vi "Main.vi"(8 "error in":errorcluster, 11 "gui in":refnum<class "gui.lvclass">) -> (0 "error out":errorcluster, 3 "gui out":refnum<class "gui.lvclass">)   [LabVIEW 2023, in "GUI.lvlib" / "gui.lvclass"]
doc: "The <b>Queued Message Handler</b> of the Worker that owns this VI."
uses:
  gui.lvclass
  C:/Program Files/National Instruments/LabVIEW 2023/vi.lib/addons/_Workers/Library/Classes/Worker/Worker.lvclass
  Pump_lvlib/TypeDef/pair_Type.ctl
  Drive/Rotation Control Type.ctl
  Pump_lvlib/TypeDef/pump_Type_Pair_L.ctl
  Pump_lvlib/TypeDef/pump_Type_Pair_R.ctl
  Pump_lvlib/TypeDef/parametrs_Type.ctl
  Modbus PLC/Modbus PLC/Data.ctl
  Modbus PLC/Modbus PLC/Commands.ctl
  gui.lvclass/gui.ctl
  Initialization Data.ctl
  Response Cases.ctl
  Settings Window/Initialization Data.ctl
  Settings Window/Response Cases.ctl
  <vilib>/addons/_Workers/Library/Case Label.ctl
  rql_Get Pumps.ctl
  rql_Push Pumps.ctl
  rqp_Open Settings.ctl
  rqp_Pumps Change.ctl
  Pump_lvlib/Pumps Worker/rqp_Write Data.ctl
  rqp_Recombination Change.ctl
  rqp_Mixer Change.ctl
  rqp_Heater Change.ctl
  rqp_Get Initialize Data.ctl
  rqp_Write CMD.ctl
  Pump_lvlib/Pumps Worker/rqp_Get Settings.ctl
  <vilib>/addons/_Workers/Library/Classes/Message/Priority.ctl
  <vilib>/addons/_Workers/Library/Classes/Message Queue/Message Queue.lvclass
  Registration Worker/Registration.lvclass
  Modbus PLC/Modbus PLC/Modbus PLC.lvclass
  Pump_lvlib/Pumps Worker/Pumps Worker.lvclass
  Settings Window/Settings Window.lvclass
  <vilib>/addons/_Workers/Library/Workers.lvlib
  Graph_data_collector/Graph_data_collector.lvlib
  Registration/Registration.lvlib
  Message Pump/Message Pump.lvclass
  Initial Data/Initial Data.lvlib
  AutoPV/AutoPV.lvlib
  Pump_lvlib/pump_Lib.lvlib
  <vilib>/addons/_Workers/Library/Classes/Message/Message.lvclass
  C:/Program Files/National Instruments/LabVIEW 2023/vi.lib/addons/_Workers/Library/Classes/Workers Object/Workers Object.lvclass
  J:/Work/Cortech/KTM 1001/Workers/gui/gui.lvclass
  GUI.lvlib
  Drive/Drive.lvlib
panel:
  in  "CurvePV Btn":bool
  in  "Registration Btn":bool
  in  "Settings Btn":bool
  in  "Camera Btn":bool
  in  "Graph Btn":bool
  in  "Скорость, об/мин":dbl format="%#_f"
  in  "Mixer Start":bool
  in  "Temp speed":dbl caption="Скорость, °С/мин" format="%#_f"
  in  "End by temperature":dbl caption="Конечная температура, °С" format="%#_f"
  in  "Temp Speed Mode":bool
  in  "Termostat":dbl caption="Термостат, °С" format="%#_f"
  in  "Heater Start Btn":bool
  in  "Current Temperature":dbl caption="Текущая температура, °С" format="%#_f"
  in  "Уставка, °С":sgl format="%#_f"
  in  "Rotate":T1={"Mode"=1, "PV Angle"=0.0, "SP_Angle"=0.0, "Rotate Angle"=0.0, "Timeout"=0.0, "Start"=FALSE, "Home"=FALSE} caption="Поворот" {"Rotate Angle" format="%.1f"; "SP_Angle" format="%.1f"; "PV Angle" format="%.2f"; "Mode" items=["Поворот"=1, "Качение"=2]}
  in  "Control Button":bool
  in  "Насосная система":T2={"Давление заданное"=0.3, "Давление в системе"=99.99, "Расход заданый"=0.0, "Расход текущий"=0.0, "Объём заданный"=0.0, "Объём текущий"=0.0, "Старт давление"=FALSE, "Старт расход"=FALSE, "Сброс объёма"=FALSE, "plc_control"=FALSE, "lag_control"=FALSE, "mstop_control"=FALSE, "Давление"={"АЦП CH 0"=0.0, "АЦП CH 1"=0.0, "АЦП CH 2"=0.0, "АЦП CH 3"=0.0, "АЦП CH 4"=0.0, "АЦП CH 5"=0.0, "АЦП CH 6"=0.0, "АЦП CH 7"=0.0}, "Modbus"={"Массив чтения"=[], "Массив записи"=[]}} {"Давление"."АЦП CH 7" format="%.3f"; "Давление"."АЦП CH 6" format="%.3f"; "Давление"."АЦП CH 5" format="%.3f"; "Давление"."АЦП CH 4" format="%.3f"; "Давление"."АЦП CH 3" format="%.3f"; "Давление"."АЦП CH 2" format="%.3f"; "Давление"."АЦП CH 1" format="%.3f"; "Давление"."АЦП CH 0" format="%.3f"; "Объём текущий" min=0.0 max=9999.0 step=0.0001 format="%#_4f"; "Объём заданный" min=0.0 max=9999.0 step=0.0001 format="%#_5f"; "Расход текущий" format="%#_4f"; "Расход заданый" min=-150.0 max=150.0 step=0.0001 format="%#_5f"; "Давление в системе" format="%.2f"; "Давление заданное" min=0.3 max=100.0 step=0.01 format="%#_5f"}
  in  "CMD":T3 {"Mix_CMD" items=["Мешалка движение вперёд"=1, "Мешалка движение назад"=2, "Мешалка стоп"=9]; "Termex_CMD" items=["Термостат старт"=1, "Термостат стоп"=9]; "Rotate_CMD" items=["Качалка Дом"=1, "Качалка Режим Авто - Старт"=2, "Качалка Режим Ручной - Старт"=3, "Качалка Стоп"=9]}
  out "data":T4 {"Rotate_IND" items=["стоп", "Качалка Режим Авто", "Качалка Режим Ручной"]; "Termex_IND" items=["Термостат старт"=1, "Термостат стоп"=0]; "Mix_IND" items=["Мешалка движение вперёд"=1, "Мешалка движение назад"=2, "Мешалка стоп"=0]}
  in  "Параметры":T5
  in  "Насос 2":T6={"Давление заданное"=0.3, "Давление MAX заданное"=100.0, "Давление в насосе"=0.0, "Давление в системе"=99.99, "Расход заданый"=0.0, "Расход текущий"=0.0, "Объём заданный"=0.0, "Объём текущий"=0.0, "Позиция насоса %"=0.0, "Ток двигателя"=0.0, "controlMsg"="", "Клапан k_sys"=FALSE, "Клапан k_res"=FALSE, "Клапан k_air"=FALSE, "Вверх"=FALSE, "Домой"=FALSE, "Вниз"=FALSE, "Старт расход"=FALSE, "Старт давление"=FALSE, "Сброс объёма"=FALSE, "Сброс давления Рсис"=FALSE, "Сброс давления Рнас"=FALSE, "Bits"={"plc_control"=FALSE, "lag_control"=FALSE, "mstop_control"=FALSE, "st_home"=FALSE, "error"=FALSE, "mstart"=FALSE, "pair"=FALSE, "startQ"=FALSE, "startP"=FALSE, "volume_Stop"=FALSE}} {"Ток двигателя" format="%#_5f"; "Расход текущий" format="%#_4f"; "Давление в системе" format="%.2f"; "Объём текущий" min=0.0 max=9999.0 step=0.0001 format="%#_4f"; "Объём заданный" min=0.0 max=9999.0 step=0.0001 format="%#_5f"; "Давление MAX заданное" min=0.0 max=100.0 step=0.01 format="%#_5f"; "Давление заданное" min=0.3 max=100.0 step=0.01 format="%#_5f"; "Расход заданый" min=-150.0 max=150.0 step=0.0001 format="%#_5f"; "Давление в насосе" format="%.3f"; "Позиция насоса %" scale=0.0..100.0 scale format="%.2f"}
  in  "Насос":T7={"Давление заданное"=0.3, "Давление MAX заданное"=100.0, "Давление в насосе"=0.0, "Давление в системе"=99.99, "Расход заданый"=0.0, "Расход текущий"=0.0, "Объём заданный"=0.0, "Объём текущий"=0.0, "Позиция насоса %"=0.0, "Ток двигателя"=0.0, "controlMsg"="", "Клапан k_sys"=FALSE, "Клапан k_res"=FALSE, "Клапан k_air"=FALSE, "Вверх"=FALSE, "Домой"=FALSE, "Вниз"=FALSE, "Старт расход"=FALSE, "Старт давление"=FALSE, "Сброс объёма"=FALSE, "Сброс давления Рсис"=FALSE, "Сброс давления Рнас"=FALSE, "Bits"={"plc_control"=FALSE, "lag_control"=FALSE, "mstop_control"=FALSE, "st_home"=FALSE, "error"=FALSE, "mstart"=FALSE, "pair"=FALSE, "startQ"=FALSE, "startP"=FALSE, "volume_Stop"=FALSE}} {"Ток двигателя" format="%#_5f"; "Расход текущий" format="%#_4f"; "Давление в системе" format="%.2f"; "Объём текущий" min=0.0 max=9999.0 step=0.0001 format="%#_4f"; "Объём заданный" min=0.0 max=9999.0 step=0.0001 format="%#_5f"; "Давление MAX заданное" min=0.0 max=100.0 step=0.01 format="%#_5f"; "Давление заданное" min=0.3 max=100.0 step=0.01 format="%#_5f"; "Расход заданый" min=-150.0 max=150.0 step=0.0001 format="%#_5f"; "Давление в насосе" format="%.3f"; "Позиция насоса %" scale=0.0..100.0 scale format="%.2f"}
  out "T ind":dbl caption="Температура, C"
  out "V ind":dbl caption="Объем, см^3"
  out "P ind":dbl caption="Давление, МПа"
  # "Насосная тележка"
  # "Рекомбинация"
  # "Мешалка"
  # "Нагрев"
  # "%"
  # "%"
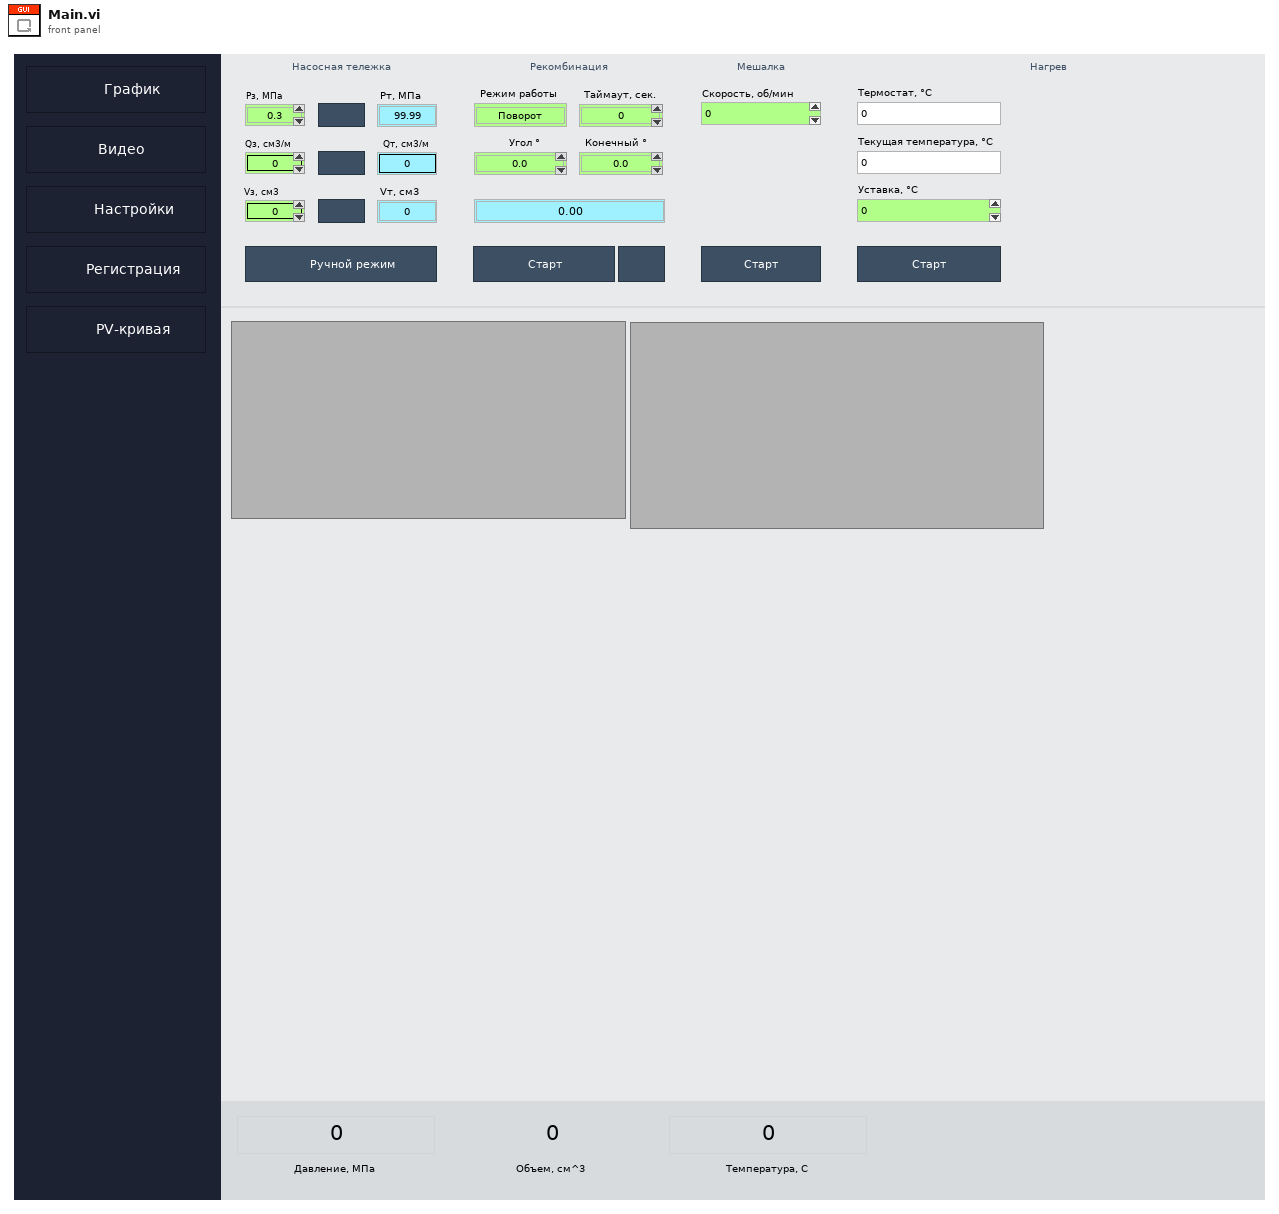
[diagram p1: front panel]
types:
  T1 = typedef "Drive.lvlib/Rotation Control Type.ctl" = cluster{"Mode":u16, "PV Angle":dbl, "SP_Angle":dbl, "Rotate Angle":dbl, "Timeout":dbl, "Start":bool, "Home":bool}
  T2 = typedef "pump_Lib.lvlib/pair_Type.ctl" = cluster{"Давление заданное":dbl, "Давление в системе":dbl, "Расход заданый":dbl, "Расход текущий":dbl, "Объём заданный":dbl, "Объём текущий":dbl, "Старт давление":bool, "Старт расход":bool, "Сброс объёма":bool, "plc_control":bool, "lag_control":bool, "mstop_control":bool, "Давление":cluster{"АЦП CH 0":dbl, "АЦП CH 1":dbl, "АЦП CH 2":dbl, "АЦП CH 3":dbl, "АЦП CH 4":dbl, "АЦП CH 5":dbl, "АЦП CH 6":dbl, "АЦП CH 7":dbl}, "Modbus":cluster{"Массив чтения":u16[], "Массив записи":u16[]}}
  T3 = typedef "Modbus PLC.lvlib/Modbus PLC.lvclass/Commands.ctl" = cluster{"Rotate_CMD":u16, "Termex_CMD":u16, "Mix_CMD":u16, "Rotate_SP_Angle_Init":u16, "Rotate_SP_Angle_End":u16, "Rotate_SP_Timeout":u16, "Rotate_SP_Speed":u16, "T_SP":sgl, "KP":sgl, "TN":sgl, "Mix_SP":u16}
  T4 = typedef "Modbus PLC.lvlib/Modbus PLC.lvclass/Data.ctl" = cluster{"Rotate_IND":u16, "Termex_IND":u16, "Mix_IND":u16, "Rotate_PV_Angle_Init":u16, "Rotate_PV_Angle_End":u16, "Rotate_PV_Timeout":u16, "Rotate_PV_Speed":u16, "Rotate_PV_Time":u16, "Rotate_PV_Angle":u16, "Termex_SP":sgl, "MIX_PV":u16, "Termex_PV_In":sgl, "Termex_KP":sgl, "P_PV":sgl, "Termex_PV_Out":sgl, "Termex_TN":sgl, "MM_PV":sgl}
  T5 = typedef "pump_Lib.lvlib/parametrs_Type.ctl" = cluster{"мл в час":bool, "Спарить насосы":bool, "DO-1":u16[]}
  T6 = typedef "pump_Lib.lvlib/pump_Type_Pair_R.ctl" = cluster{"Давление заданное":dbl, "Давление MAX заданное":dbl, "Давление в насосе":dbl, "Давление в системе":dbl, "Расход заданый":dbl, "Расход текущий":dbl, "Объём заданный":dbl, "Объём текущий":dbl, "Позиция насоса %":dbl, "Ток двигателя":dbl, "controlMsg":string, "Клапан k_sys":bool, "Клапан k_res":bool, "Клапан k_air":bool, "Вверх":bool, "Домой":bool, "Вниз":bool, "Старт расход":bool, "Старт давление":bool, "Сброс объёма":bool, "Сброс давления Рсис":bool, "Сброс давления Рнас":bool, "Bits":cluster{"plc_control":bool, "lag_control":bool, "mstop_control":bool, "st_home":bool, "error":bool, "mstart":bool, "pair":bool, "startQ":bool, "startP":bool, "volume_Stop":bool}}
  T7 = typedef "pump_Lib.lvlib/pump_Type_Pair_L.ctl" = cluster{"Давление заданное":dbl, "Давление MAX заданное":dbl, "Давление в насосе":dbl, "Давление в системе":dbl, "Расход заданый":dbl, "Расход текущий":dbl, "Объём заданный":dbl, "Объём текущий":dbl, "Позиция насоса %":dbl, "Ток двигателя":dbl, "controlMsg":string, "Клапан k_sys":bool, "Клапан k_res":bool, "Клапан k_air":bool, "Вверх":bool, "Домой":bool, "Вниз":bool, "Старт расход":bool, "Старт давление":bool, "Сброс объёма":bool, "Сброс давления Рсис":bool, "Сброс давления Рнас":bool, "Bits":cluster{"plc_control":bool, "lag_control":bool, "mstop_control":bool, "st_home":bool, "error":bool, "mstart":bool, "pair":bool, "startQ":bool, "startP":bool, "volume_Stop":bool}}
  T8 = typedef "Initial Data.lvlib/Broadcast Events--cluster.ctl" = cluster{"Module Did Init":refnum<user-event>, "Status Updated":refnum<user-event>, "Error Reported":refnum<user-event>, "Module Did Stop":refnum<user-event>, "Update Module Execution Status":refnum<user-event>, "Data":refnum<user-event>}
  T9 = typedef "Registration.lvlib/Broadcast Events--cluster.ctl" = cluster{"Module Did Init":refnum<user-event>, "Status Updated":refnum<user-event>, "Error Reported":refnum<user-event>, "Module Did Stop":refnum<user-event>, "Update Module Execution Status":refnum<user-event>, "Data from Registration":refnum<user-event>, "Get Main VI Reference":refnum<user-event>}
  T10 = typedef "Settings Window.lvclass/Initialization Data.ctl" = cluster{"Response Cases":T11, "Config Path":path}
  T11 = typedef "Settings Window.lvclass/Response Cases.ctl" = cluster{"Placeholder - Can be deleted":string, "Get Settings":T12, "Starting Settings":T12}
  T12 = typedef "Workers.lvlib/Case Label.ctl" = string
  T13 = typedef "GUI.lvlib/gui.lvclass/Initialization Data.ctl" = cluster{"Response Cases":T14}
  T14 = typedef "GUI.lvlib/gui.lvclass/Response Cases.ctl" = cluster{"Placeholder - Can be deleted":string}
  T15 = typedef "GUI.lvlib/gui.lvclass/rql_Get Pumps.ctl" = cluster{"String":string}
  T16 = typedef "GUI.lvlib/gui.lvclass/rql_Push Pumps.ctl" = cluster{"String":string}
  T17 = typedef "GUI.lvlib/gui.lvclass/rqp_Open Settings.ctl" = cluster{"String":string}
  T18 = typedef "pump_Lib.lvlib/Pumps Worker.lvclass/rqp_Write Data.ctl" = cluster{"Насос":T7, "Насос 2":T6, "Насосная система":T2}
  T19 = typedef "GUI.lvlib/gui.lvclass/rqp_Pumps Change.ctl" = cluster{"String":string}
  T20 = typedef "GUI.lvlib/gui.lvclass/rqp_Recombination Change.ctl" = cluster{"String":string}
  T21 = typedef "GUI.lvlib/gui.lvclass/rqp_Mixer Change.ctl" = cluster{"String":string}
  T22 = typedef "GUI.lvlib/gui.lvclass/rqp_Heater Change.ctl" = cluster{"String":string}
  T23 = typedef "GUI.lvlib/gui.lvclass/rqp_Get Initialize Data.ctl" = cluster{"Дата":string, "Время":string, "Месторождение":string, "Пласт":string, "Скважина":string}
  T24 = typedef "GUI.lvlib/gui.lvclass/rqp_Write CMD.ctl" = cluster{"CMD":T3}
  T25 = typedef "pump_Lib.lvlib/Pumps Worker.lvclass/rqp_Get Settings.ctl" = cluster{"Pump":refnum<vi>, "Params":refnum<vi>, "Pump2":refnum<vi>, "Pump System":refnum<vi>, "IP Adress":string}
  T26 = typedef "Workers.lvlib/Message.lvclass/Priority.ctl" = enum16{"Low", "Normal", "High"}
  T27 = enum8{"Enabled", "Disabled", "Disabled and Grayed Out"}
  T28 = typedef "pump_Lib.lvlib/pump_Type.ctl" = cluster{"Давление заданное":dbl, "Давление MAX заданное":dbl, "Давление в насосе":dbl, "Давление в системе":dbl, "Расход заданый":dbl, "Расход текущий":dbl, "Объём заданный":dbl, "Объём текущий":dbl, "Позиция насоса %":dbl, "Ток двигателя":dbl, "controlMsg":string, "Клапан k_sys":bool, "Клапан k_res":bool, "Клапан k_air":bool, "Вверх":bool, "Домой":bool, "Вниз":bool, "Старт расход":bool, "Старт давление":bool, "Сброс объёма":bool, "Сброс давления Рсис":bool, "Сброс давления Рнас":bool, "Bits":cluster{"plc_control":bool, "lag_control":bool, "mstop_control":bool, "st_home":bool, "error":bool, "mstart":bool, "pair":bool, "startQ":bool, "startP":bool, "volume_Stop":bool}}
  T29 = typedef "Settings Window.lvclass/rsp_Get Settings.ctl" = cluster{"Settings":T30}
  T30 = typedef "Settings Window.lvclass/Settings.ctl" = cluster{"PLC1":cluster{"port":u16, "address":string}, "PLC2":cluster{"port":u16, "address":string}, "Heater":cluster{"P":dbl, "I":dbl}, "Calcs":cluster{"Vm0":dbl, "K0":dbl, "a_small":dbl, "A":dbl, "b_small":dbl, "B":dbl}}
  T31 = typedef "pump_Lib.lvlib/Pumps Worker.lvclass/rsp_New Pumps Data.ctl" = cluster{"Насос":T7, "Насос 2":T6, "Насосная система":T2}
  T32 = typedef "Settings Window.lvclass/rsp_Starting Settings.ctl" = cluster{"Settings":T30}
  T33 = cluster{"Vm0":dbl, "K0":dbl, "a_small":dbl, "A":dbl, "b_small":dbl, "B":dbl}
  T34 = typedef "Registration.lvclass/rsp_Record Status to Caller.ctl" = bool
  T35 = typedef "Initial Data.lvlib/InitalData Type.ctl" = cluster{"Дата":string, "Время":string, "Месторождение":string, "Пласт":string, "Скважина":string}
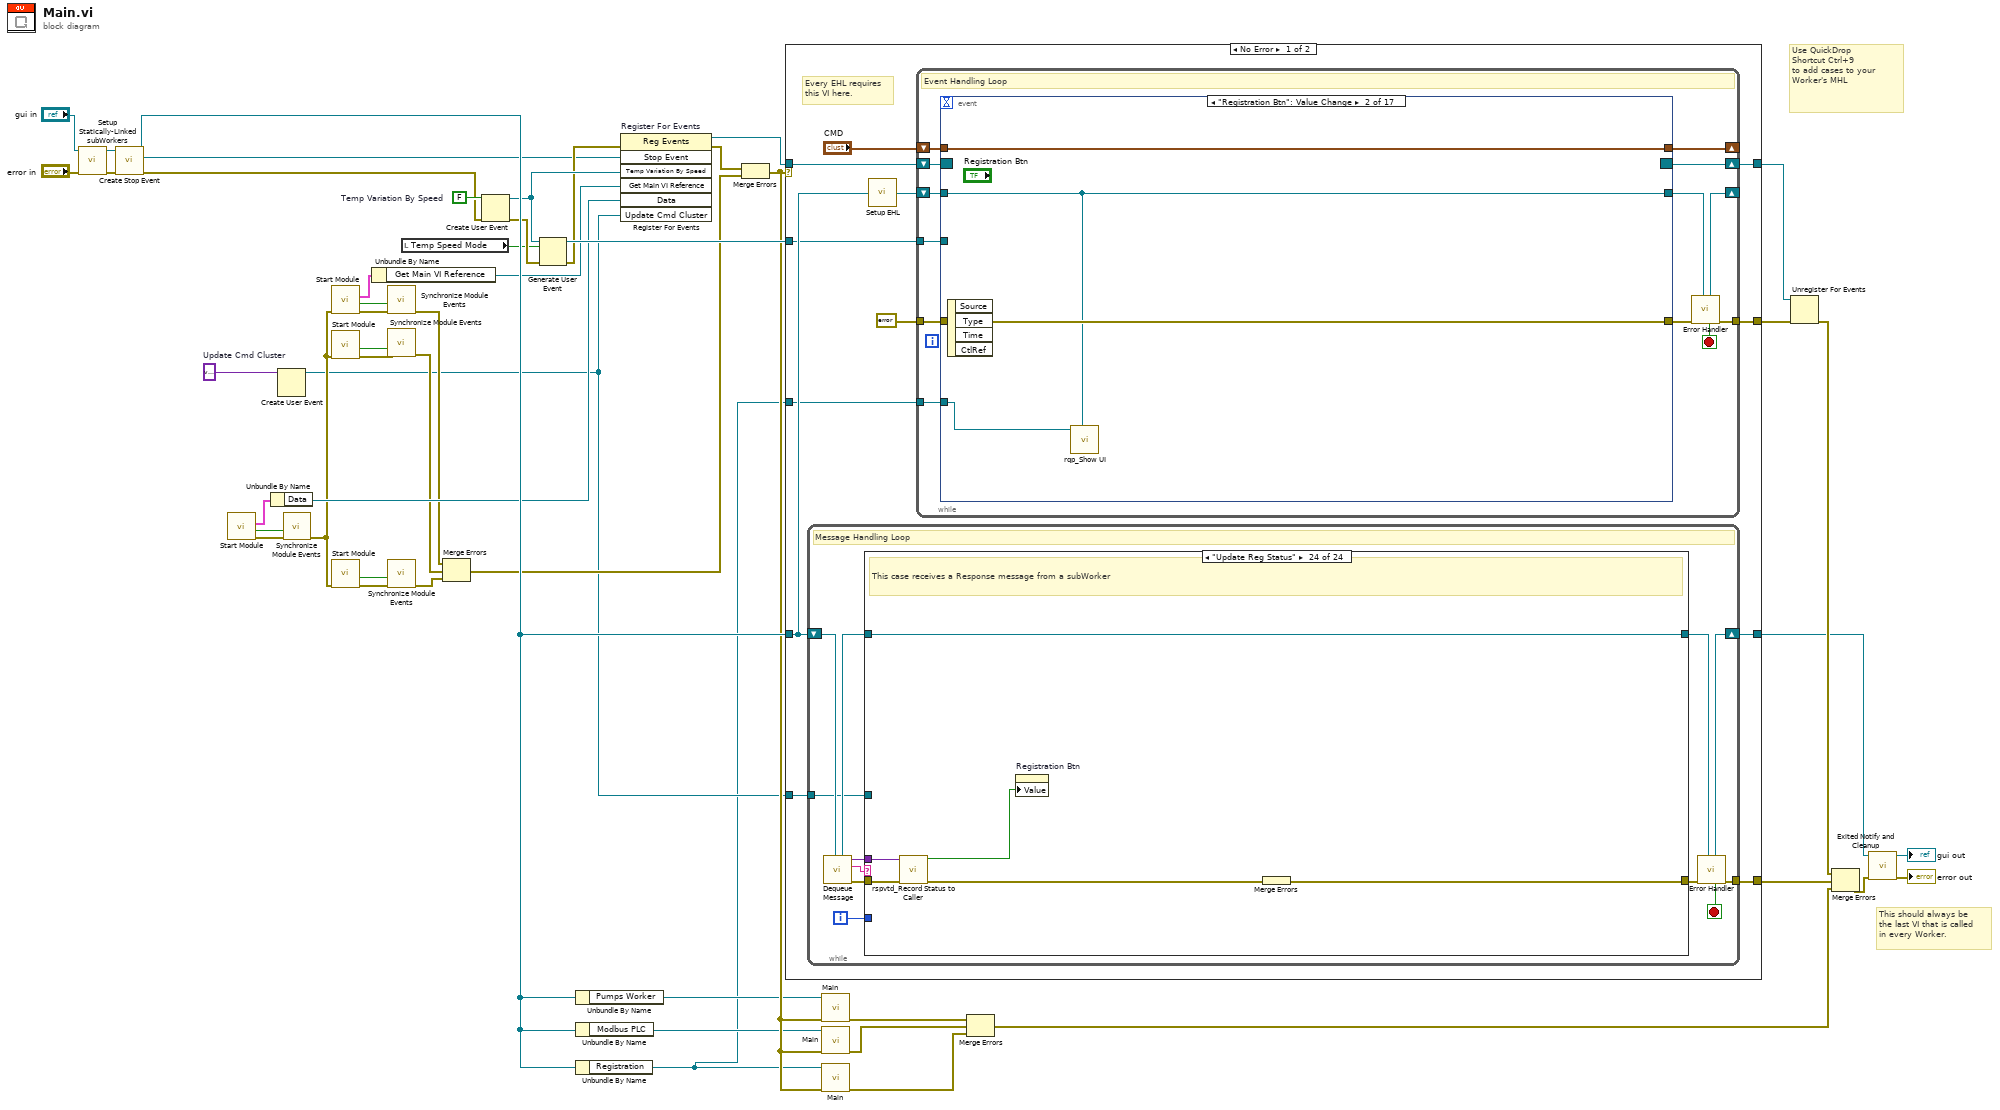
[diagram p0: block diagram]
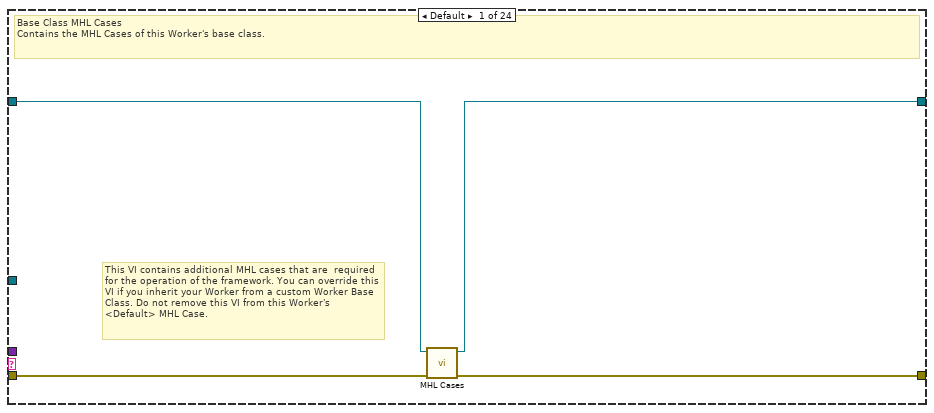
[diagram p2: hidden frame]
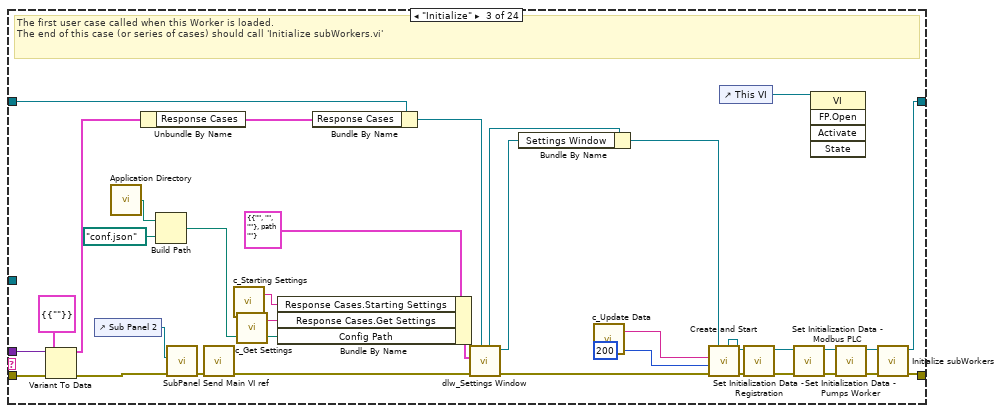
[diagram p4: hidden frame]
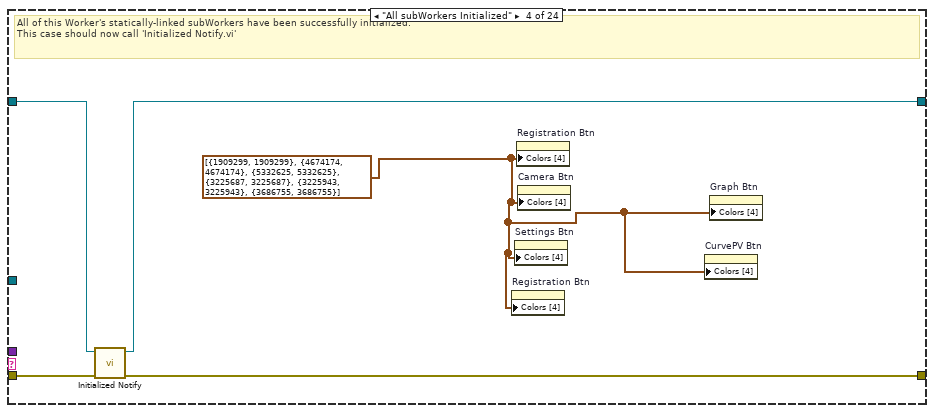
[diagram p5: hidden frame]
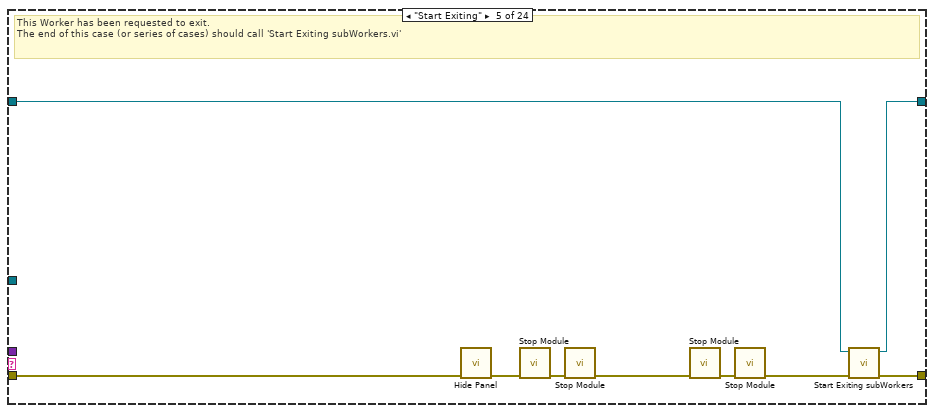
[diagram p6: hidden frame]
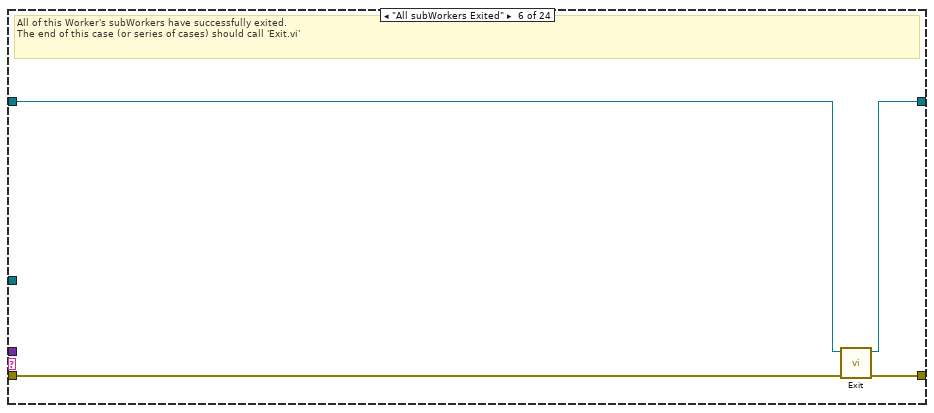
[diagram p7: hidden frame]
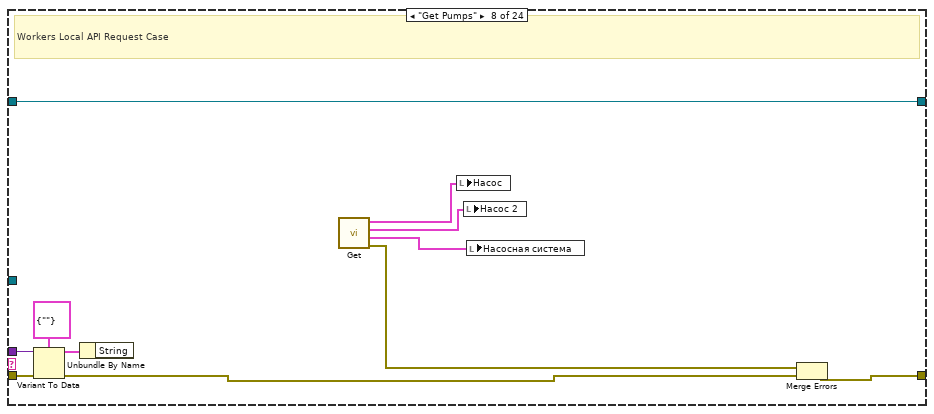
[diagram p9: hidden frame]
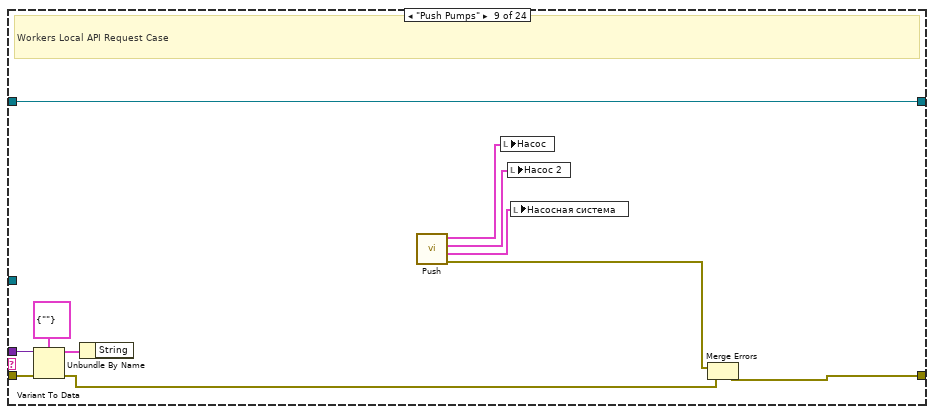
[diagram p10: hidden frame]
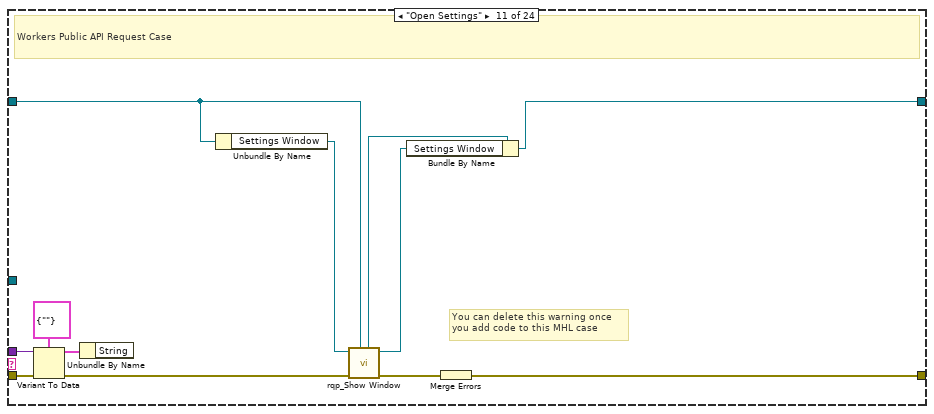
[diagram p12: hidden frame]
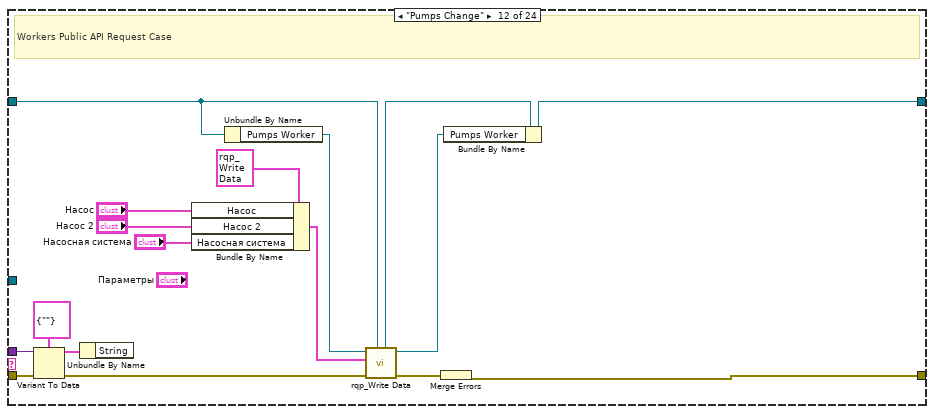
[diagram p13: hidden frame]
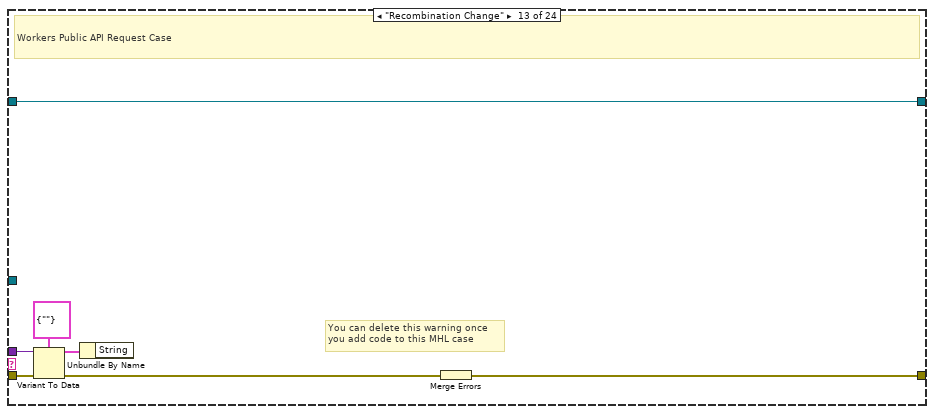
[diagram p14: hidden frame]
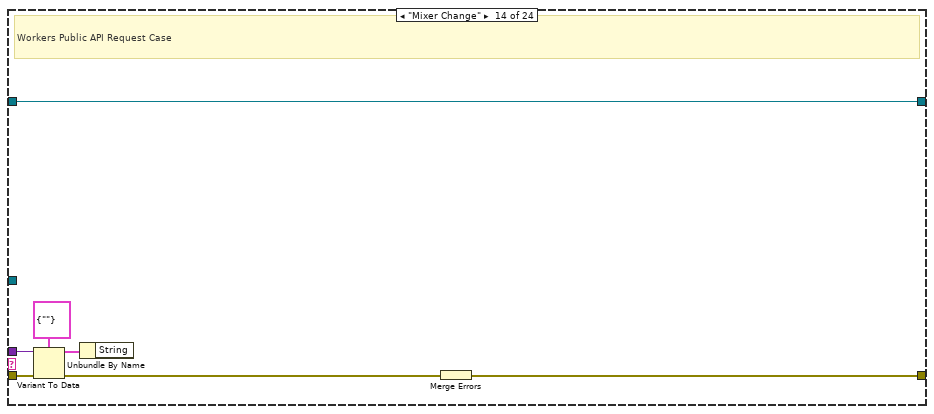
[diagram p15: hidden frame]
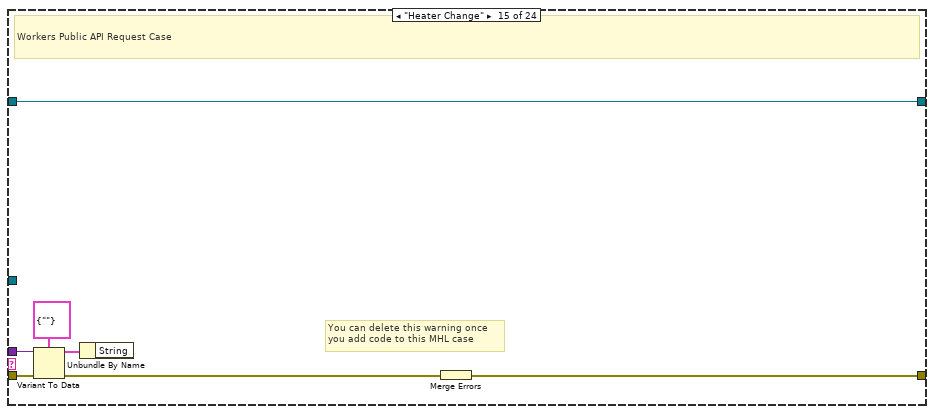
[diagram p16: hidden frame]
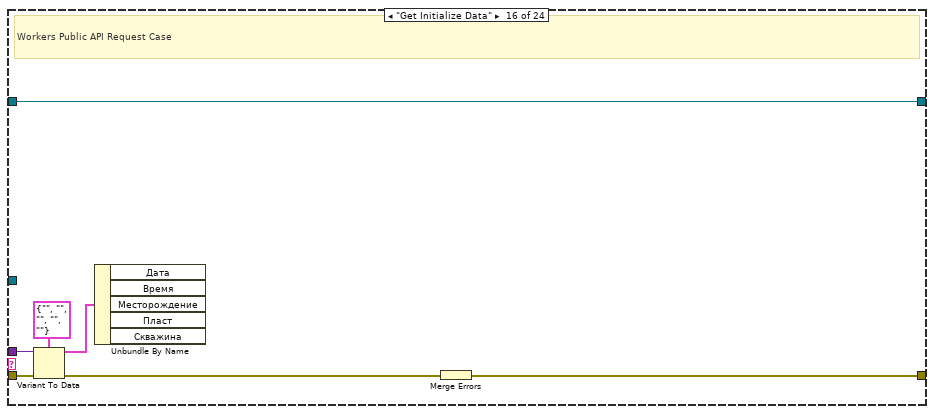
[diagram p17: hidden frame]
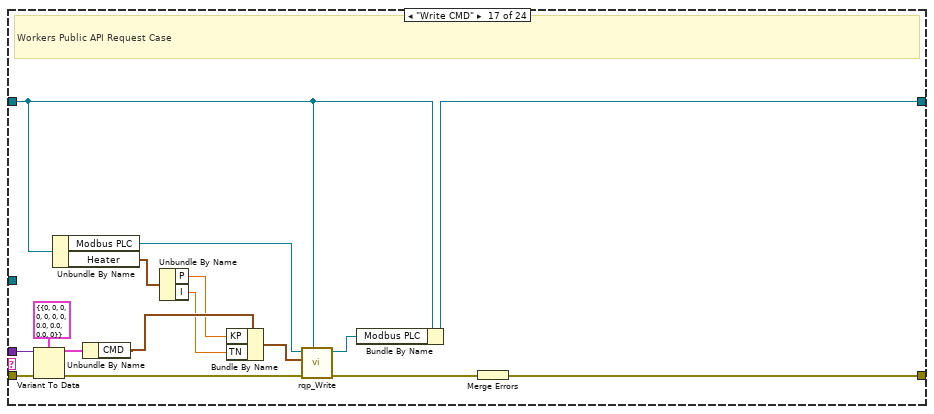
[diagram p18: hidden frame]
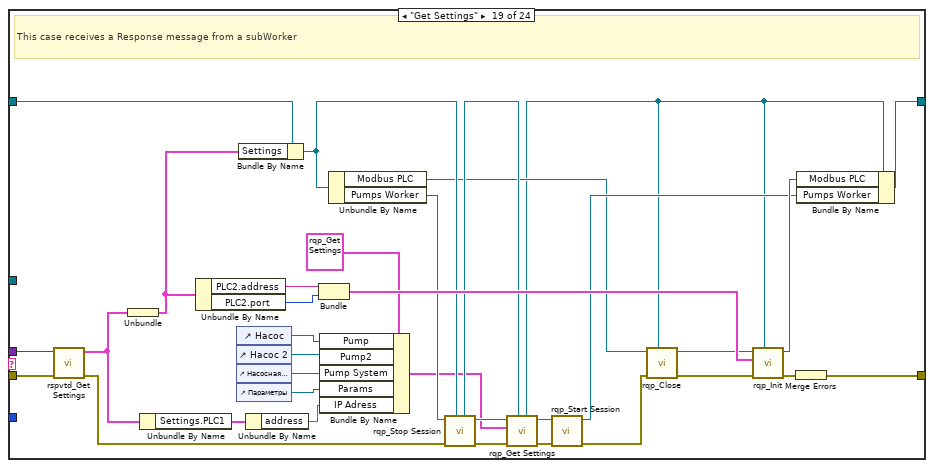
[diagram p20: hidden frame]
diagram:
  w4 = variant  # Update Cmd Cluster
  w40 = FALSE  # Temp Variation By Speed
  # "Use QuickDrop\nShortcut Ctrl+9\nto add cases to your\nWorker's MHL"
  # "This should always be the last VI that is called in every Worker."
  n1 = call "Setup Statically-Linked subWorkers.vi"("error in"="error in", "gui in"="gui in") -> ("error out"=w13:errorcluster, "gui out"=w11:refnum<class "gui.lvclass">)  [unwired: 8 in]
  n2 = call-dynamic "Create Stop Event.vi"("error in"=w13, "Worker"=w11) -> ("error out"=w39:errorcluster, "Stop Event"=w14:refnum<user-event>, "Worker out"=w42:refnum<class "gui.lvclass">)  [unwired: 7 in]
  n3 = call "Start Module.vi"() -> ("error out"=w25:errorcluster, "Wait for Event Sync?"=w24:bool, "Initial Data Broadcast Events"=w27:T8)  [unwired: 8 in, 1 out]
  n4 = Unbundle By Name(w27) -> ("Data"=w26:refnum<user-event>)
  n5 = Create User Event(user event datatype=w4) -> (user event=w3:refnum<user-event>)  [unwired: 1 in, 1 out]
  n6 = call "Synchronize Module Events.vi"("error in"=w25, "Wait for Event Sync?"=w24) -> ("error out"=w15:errorcluster)  [unwired: 9 in]
  n7 = call "Start Module.vi"("error in"=w15) -> ("error out"=w32:errorcluster, "Wait for Event Sync?"=w31:bool, "Registration Broadcast Events"=w33:T9)  [unwired: 7 in, 1 out]
  n8 = call "Start Module.vi"("error in"=w15) -> ("error out"=w29:errorcluster, "Wait for Event Sync?"=w30:bool)  [unwired: 7 in, 2 out]
  n9 = call "Start Module.vi"("error in"=w15) -> ("error out"=w23:errorcluster, "Wait for Event Sync?"=w22:bool)  [unwired: 7 in, 2 out]
  n10 = Unbundle By Name(w33) -> ("Get Main VI Reference"=w28:refnum<user-event>)
  n11 = call "Synchronize Module Events.vi"("error in"=w32, "Wait for Event Sync?"=w31) -> ("error out"=w19:errorcluster)  [unwired: 9 in]
  n12 = call "Synchronize Module Events.vi"("error in"=w29, "Wait for Event Sync?"=w30) -> ("error out"=w20:errorcluster)  [unwired: 9 in]
  n13 = call "Synchronize Module Events.vi"("error in"=w23, "Wait for Event Sync?"=w22) -> ("error out"=w21:errorcluster)  [unwired: 9 in]
  n14 = local read "Temp Speed Mode"() -> (w36:bool)
  n15 = Merge Errors(w19, w20, w21) -> (w16:errorcluster)
  n16 = Create User Event(user event datatype=w40, error in=w39) -> (user event=w37:refnum<user-event>, error out=w38:errorcluster)
  n17 = Generate User Event(user event=w37, event data cluster=w36, error in=w38) -> (user event out=w35:refnum<user-event>, error out=w34:errorcluster)  [unwired: 1 in]
  n18 = Unbundle By Name(w42) -> ("Pumps Worker"=w8:refnum<class "Pumps Worker.lvclass">)
  n19 = Unbundle By Name(w42) -> ("Modbus PLC"=w6:refnum<class "Modbus PLC.lvclass">)
  n20 = Unbundle By Name(w42) -> ("Registration"=w1:refnum<class "Registration.lvclass">)
  n21 = register-events "Register For Events"(error in=w34, w14, w37, w28, w26, w3) -> (reference out=w5:refnum<event-registration>, error out=w18:errorcluster)  [unwired: 1 in]
  n22 = Merge Errors(w18, w16) -> (w17:errorcluster)
  n23 = case shown="No Error" w17 {
    tunnel: w42 -> [w57 w519]
    tunnel: [w55 w520] -> w45
    tunnel: w5 -> [w62 w521]
    tunnel: [w59 w522] -> w49
    tunnel: [w61 w521] -> w48
    tunnel: [w56 w518] -> w46
    selector: w17 -> [_ w522]
    tunnel: w35 -> [w54 _]
    tunnel: w3 -> [w52 _]
    tunnel: w1 -> [w51 _]
    frame No Error {
      # "Every EHL requires\nthis VI here."
      n24 = while {
        shift-right: [w72] -> w56
        shift-left: w57 -> [w74]
        tunnel: [w73] -> w55
        tunnel: w52 -> [w63]
        i -> [w65]
        stop <- w66 stop-if-true
        # "Message Handling Loop"
        n25 = call-dynamic "Dequeue Message.vi"("Worker"=w74) -> ("error out"=w71:errorcluster, "Case out"=w67:string, "Data out"=w64:variant, "Worker out"=w69:refnum<class "gui.lvclass">)  [unwired: 6 in, 1 out]
        n26 = case "Worker MHL Case Structure (DO NOT CHANGE LABEL NAME)" shown="\"Update Reg Status\"" w67 {
          tunnel: w71 -> [w78 w79 w113 w118 w122 w133 w135 w146 w156 w159 w171 w188 w194 w201 w208 w215 w232 w234 w266 w272 w279 w309 w334 w339]
          tunnel: [w77 w79 w115 w117 w129 w132 w135 w141 w151 w159 w167 w184 w189 w196 w203 w210 w228 w234 w268 w270 w273 w282 w335 w340] -> w70
          tunnel: w69 -> [w76 w80 w112 w120 w127 w131 w134 w136 w157 w158 w164 w180 w195 w202 w209 w216 w225 w233 w265 w271 w281 w305 w330 w341]
          tunnel: [w75 w80 w114 w119 w128 w130 w134 w136 w157 w158 w160 w177 w195 w202 w209 w216 w223 w233 w261 w271 w281 w304 w330 w341] -> w68
          tunnel: w65 -> [_ _ _ _ _ _ _ _ _ _ _ _ _ _ _ _ _ _ _ _ _ _ _ _]
          tunnel: w64 -> [_ _ w111 _ _ _ _ w143 w153 _ w169 w186 w191 w198 w205 w212 w230 _ w267 _ w280 w308 w331 w337]
          tunnel: w63 -> [_ _ _ _ _ _ _ _ _ _ _ _ _ _ _ _ _ _ _ _ _ _ w313 _]
          frame Default {
            # "This VI contains additional MHL cases that are  required for the operation of the framework. You can override this VI if you inherit your Worker from a custom Worker Base Class. Do not remove this VI from this Worker's <Default> MHL Case."
            # "Base Class MHL Cases\nContains the MHL Cases of this Worker's base class."
            n27 = call-dynamic "MHL Cases.vi"("error in"=w78, "Worker in"=w76) -> ("error out"=w77:errorcluster, "Worker out"=w75:refnum<class "gui.lvclass">)  [unwired: 8 in]
          }
          frame "------------ FRAMEWORK CASES -----------" {
            # "Start of Workers Framework Cases"
          }
          frame "Initialize" {
            # "The first user case called when this Worker is loaded.\nThe end of this case (or series of cases) should call 'Initialize subWorkers.vi'"
            n28 = Variant To Data(error in=w113, type=T13 {"Response Cases"={"Placeholder - Can be deleted"=""}} ("Initialization Data"), Variant=w111) -> (data=w110:T13, error out=w103:errorcluster)
            n29 = control-ref of="Sub Panel 2"() -> (w105:refnum<vi>)
            n30 = call <vilib>:"Application Directory.vi"() -> ("Application Directory"=w91:path)
            n31 = Unbundle By Name(w110) -> ("Response Cases"=w109:T14)
            n32 = Build Path(base path=w91, name or relative path=path "conf.json") -> (appended path=w89:path)
            n33 = call "SubPanel.vi"("error in"=w103, "Sub Panel"=w105) -> ("error out"=w104:errorcluster)  [unwired: 9 in]
            n34 = call "Send Main VI ref.vi"("error in"=w104) -> ("error out"=w99:errorcluster)  [unwired: 10 in]
            n35 = call "c_Starting Settings.vi"() -> ("Case Label"=w88:T12)  [unwired: 1 in]
            n36 = call "c_Get Settings.vi"() -> ("Case Label"=w101:T12)  [unwired: 1 in]
            n37 = Bundle By Name(cluster=T10 {"Response Cases"={"Placeholder - Can be deleted"="", "Get Settings"="", "Starting Settings"=""}, "Config Path"=path ""} ("Initialization Data"), "Response Cases.Starting Settings"=w88, "Response Cases.Get Settings"=w101, "Config Path"=w89) -> (w102:T10)
            n38 = Bundle By Name(cluster=w112, "Response Cases"=w109) -> (w97:refnum<class "gui.lvclass">)
            n39 = call "dlw_Settings Window.vi"("Caller in"=w97, "error in"=w99, "Initialization Data"=w102) -> ("error out"=w98:errorcluster, "Settings Window out"=w95:refnum<class "Settings Window.lvclass">, "dup Caller out"=w96:refnum<class "gui.lvclass">)  [unwired: 6 in]
            n40 = Bundle By Name(cluster=w96, "Settings Window"=w95) -> (w94:refnum<class "gui.lvclass">)
            n41 = call "c_Update Data.vi"() -> ("Case Label"=w106:T12)  [unwired: 1 in]
            n42 = call "Create and Start.vi"("Caller"=w94, "error in (no error)"=w98, "Period (ms)"=200, "Time Elapsed Response Case (Case Label)"=w106) -> ("error out"=w85:errorcluster, "dup Caller out"=w82:refnum<class "gui.lvclass">)  [unwired: 5 in, 1 out]
            n43 = control-ref of="This VI"() -> (w84:refnum<vi>)
            n44 = call "Set Initialization Data - Registration.vi"("error in"=w85, "gui in"=w82) -> ("error out"=w83:errorcluster, "gui out"=w81:refnum<class "gui.lvclass">)  [unwired: 8 in]
            n45 = call "Set Initialization Data - Modbus PLC.vi"("error in"=w83, "gui in"=w81) -> ("error out"=w87:errorcluster, "gui out"=w86:refnum<class "gui.lvclass">)  [unwired: 8 in]
            n46 = invoke class="VI" method="FP.Open"(reference=w84) -> ()  [unwired: 4 in, 5 out]
            n47 = call "Set Initialization Data - Pumps Worker.vi"("error in"=w87, "gui in"=w86) -> ("error out"=w93:errorcluster, "gui out"=w92:refnum<class "gui.lvclass">)  [unwired: 8 in]
            n48 = call-dynamic "Initialize subWorkers.vi"("error in"=w93, "Worker"=w92) -> ("error out"=w115:errorcluster, "dup Worker out"=w114:refnum<class "gui.lvclass">)  [unwired: 8 in]
          }
          frame "All subWorkers Initialized" {
            w116 = cluster{u32, u32}[] [{1909299, 1909299}, {4674174, 4674174}, {5332625, 5332625}, {3225687, 3225687}, {3225943, 3225943}, {3686755, 3686755}] ("Colors [4]")
            # "All of this Worker's statically-linked subWorkers have been successfully initialized.\nThis case should now call 'Initialized Notify.vi'"
            n49 = call-dynamic "Initialized Notify.vi"("error in"=w118, "Worker"=w120) -> ("error out"=w117:errorcluster, "dup Worker out"=w119:refnum<class "gui.lvclass">)  [unwired: 8 in]
            n50 = property on="Registration Btn" class="Bool"("Colors [4]"=w116) -> ()  [unwired: 2 in, 2 out]
            n51 = property on="Settings Btn" class="Bool (strict)"("Colors [4]"=w116) -> ()  [unwired: 2 in, 2 out]
            n52 = property on="Registration Btn" class="Bool"("Colors [4]"=w116) -> ()  [unwired: 2 in, 2 out]
            n53 = property on="Camera Btn" class="Bool (strict)"("Colors [4]"=w116) -> ()  [unwired: 2 in, 2 out]
            n54 = property on="CurvePV Btn" class="Bool (strict)"("Colors [4]"=w116) -> ()  [unwired: 2 in, 2 out]
            n55 = property on="Graph Btn" class="Bool (strict)"("Colors [4]"=w116) -> ()  [unwired: 2 in, 2 out]
          }
          frame "Start Exiting" {
            # "This Worker has been requested to exit. \nThe end of this case (or series of cases) should call 'Start Exiting subWorkers.vi'"
            n56 = call "Hide Panel.vi"("error in (no error)"=w122) -> ("error out"=w121:errorcluster)  [unwired: 10 in]
            n57 = call "Stop Module.vi"("error in"=w121) -> ("error out"=w126:errorcluster)  [unwired: 10 in]
            n58 = call "Stop Module.vi"("error in"=w126) -> ("error out"=w125:errorcluster)  [unwired: 10 in]
            n59 = call "Stop Module.vi"("error in"=w125) -> ("error out"=w124:errorcluster)  [unwired: 10 in]
            n60 = call "Stop Module.vi"("error in"=w124) -> ("error out"=w123:errorcluster)  [unwired: 10 in]
            n61 = call-dynamic "Start Exiting subWorkers.vi"("error_in"=w123, "Worker"=w127) -> ("error out"=w129:errorcluster, "dup Worker out"=w128:refnum<class "gui.lvclass">)  [unwired: 8 in]
          }
          frame "All subWorkers Exited" {
            # "All of this Worker's subWorkers have successfully exited. \nThe end of this case (or series of cases) should call 'Exit.vi'"
            n62 = call-dynamic "Exit.vi"("error_in"=w133, "Worker"=w131) -> ("error out"=w132:errorcluster, "dup Worker out"=w130:refnum<class "gui.lvclass">)  [unwired: 8 in]
          }
          frame "------------- LOCAL API CASES -------------" {
            # "Start of Workers Local API Cases"
          }
          frame "Get Pumps" {
            # "Workers Local API Request Case"
            n63 = Variant To Data(error in=w146, type=T15 {"String"=""} ("Data"), Variant=w143) -> (data=w142:T15, error out=w145:errorcluster)
            n64 = Unbundle By Name(w142) -> ()  [unwired: 1 out]
            n65 = call "Get.vi"() -> ("error out"=w140:errorcluster, "Pair out"=w137:T2, "Port 2 out"=w138:T28, "Port 1 out"=w139:T28)  [unwired: 8 in]
            n66 = local write "Насос"(w139) -> ()
            n67 = local write "Насос 2"(w138) -> ()
            n68 = local write "Насосная система"(w137) -> ()
            n69 = Merge Errors(w140, w145) -> (w141:errorcluster)
          }
          frame "Push Pumps" {
            # "Workers Local API Request Case"
            n70 = Variant To Data(error in=w156, type=T16 {"String"=""} ("Data"), Variant=w153) -> (data=w152:T16, error out=w155:errorcluster)
            n71 = Unbundle By Name(w152) -> ()  [unwired: 1 out]
            n72 = call "Push.vi"() -> ("error out"=w150:errorcluster, "Pair out"=w147:T2, "Port 2 out"=w148:T28, "Port 1 out"=w149:T28)  [unwired: 8 in]
            n73 = local write "Насос"(w149) -> ()
            n74 = local write "Насос 2"(w148) -> ()
            n75 = local write "Насосная система"(w147) -> ()
            n76 = Merge Errors(w150, w155) -> (w151:errorcluster)
          }
          frame "------------- PUBLIC API CASES -------------" {
            # "Start of Workers Public API Cases"
          }
          frame "Open Settings" {
            # "You can delete this warning once\nyou add code to this MHL case"
            # "Workers Public API Request Case"
            n77 = Variant To Data(error in=w171, type=T17 {"String"=""} ("Data"), Variant=w169) -> (data=w168:T17, error out=w166:errorcluster)
            n78 = Unbundle By Name(w168) -> ()  [unwired: 1 out]
            n79 = Unbundle By Name(w164) -> ("Settings Window"=w163:refnum<class "Settings Window.lvclass">)
            n80 = call "rqp_Show Window.vi"("Caller in"=w164, "error in"=w166, "Settings Window in"=w163) -> ("error out"=w165:errorcluster, "dup Settings Window out"=w161:refnum<class "Settings Window.lvclass">, "dup Caller out"=w162:refnum<class "gui.lvclass">)  [unwired: 6 in]
            n81 = Bundle By Name(cluster=w162, "Settings Window"=w161) -> (w160:refnum<class "gui.lvclass">)
            n82 = Merge Errors(w165) -> (w167:errorcluster)
          }
          frame "Pumps Change" {
            # "Workers Public API Request Case"
            n83 = Variant To Data(error in=w188, type=T19 {"String"=""} ("Data"), Variant=w186) -> (data=w185:T19, error out=w183:errorcluster)
            n84 = Unbundle By Name(w185) -> ()  [unwired: 1 out]
            n85 = Bundle By Name(cluster=T18 {"Насос"={"Давление заданное"=0.3, "Давление MAX заданное"=100.0, "Давление в насосе"=0.0, "Давление в системе"=99.99, "Расход заданый"=0.0, "Расход текущий"=0.0, "Объём заданный"=0.0, "Объём текущий"=0.0, "Позиция насоса %"=0.0, "Ток двигателя"=0.0, "controlMsg"="", "Клапан k_sys"=FALSE, "Клапан k_res"=FALSE, "Клапан k_air"=FALSE, "Вверх"=FALSE, "Домой"=FALSE, "Вниз"=FALSE, "Старт расход"=FALSE, "Старт давление"=FALSE, "Сброс объёма"=FALSE, "Сброс давления Рсис"=FALSE, "Сброс давления Рнас"=FALSE, "Bits"={"plc_control"=FALSE, "lag_control"=FALSE, "mstop_control"=FALSE, "st_home"=FALSE, "error"=FALSE, "mstart"=FALSE, "pair"=FALSE, "startQ"=FALSE, "startP"=FALSE, "volume_Stop"=FALSE}}, "Насос 2"={"Давление заданное"=0.3, "Давление MAX заданное"=100.0, "Давление в насосе"=0.0, "Давление в системе"=99.99, "Расход заданый"=0.0, "Расход текущий"=0.0, "Объём заданный"=0.0, "Объём текущий"=0.0, "Позиция насоса %"=0.0, "Ток двигателя"=0.0, "controlMsg"="", "Клапан k_sys"=FALSE, "Клапан k_res"=FALSE, "Клапан k_air"=FALSE, "Вверх"=FALSE, "Домой"=FALSE, "Вниз"=FALSE, "Старт расход"=FALSE, "Старт давление"=FALSE, "Сброс объёма"=FALSE, "Сброс давления Рсис"=FALSE, "Сброс давления Рнас"=FALSE, "Bits"={"plc_control"=FALSE, "lag_control"=FALSE, "mstop_control"=FALSE, "st_home"=FALSE, "error"=FALSE, "mstart"=FALSE, "pair"=FALSE, "startQ"=FALSE, "startP"=FALSE, "volume_Stop"=FALSE}}, "Насосная система"={"Давление заданное"=0.3, "Давление в системе"=99.99, "Расход заданый"=0.0, "Расход текущий"=0.0, "Объём заданный"=0.0, "Объём текущий"=0.0, "Старт давление"=FALSE, "Старт расход"=FALSE, "Сброс объёма"=FALSE, "plc_control"=FALSE, "lag_control"=FALSE, "mstop_control"=FALSE, "Давление"={"АЦП CH 0"=0.0, "АЦП CH 1"=0.0, "АЦП CH 2"=0.0, "АЦП CH 3"=0.0, "АЦП CH 4"=0.0, "АЦП CH 5"=0.0, "АЦП CH 6"=0.0, "АЦП CH 7"=0.0}, "Modbus"={"Массив чтения"=[], "Массив записи"=[]}}} ("Data in"), "Насос"="Насос", "Насос 2"="Насос 2", "Насосная система"="Насосная система") -> (w172:T18)
            n86 = Unbundle By Name(w180) -> ("Pumps Worker"=w179:refnum<class "Pumps Worker.lvclass">)
            n87 = call "rqp_Write Data.vi"("Caller in"=w180, "error in"=w183, "Data in"=w172, "Pumps Worker in"=w179) -> ("error out"=w182:errorcluster, "dup Pumps Worker out"=w178:refnum<class "Pumps Worker.lvclass">, "dup Caller out"=w181:refnum<class "gui.lvclass">)  [unwired: 5 in]
            n88 = Merge Errors(w182) -> (w184:errorcluster)
            n89 = Bundle By Name(cluster=w181, "Pumps Worker"=w178) -> (w177:refnum<class "gui.lvclass">)
          }
          frame "Recombination Change" {
            # "You can delete this warning once\nyou add code to this MHL case"
            # "Workers Public API Request Case"
            n90 = Variant To Data(error in=w194, type=T20 {"String"=""} ("Data"), Variant=w191) -> (data=w190:T20, error out=w193:errorcluster)
            n91 = Unbundle By Name(w190) -> ()  [unwired: 1 out]
            n92 = Merge Errors(w193) -> (w189:errorcluster)
          }
          frame "Mixer Change" {
            # "Workers Public API Request Case"
            n93 = Variant To Data(error in=w201, type=T21 {"String"=""} ("Data"), Variant=w198) -> (data=w197:T21, error out=w200:errorcluster)
            n94 = Unbundle By Name(w197) -> ()  [unwired: 1 out]
            n95 = Merge Errors(w200) -> (w196:errorcluster)
          }
          frame "Heater Change" {
            # "You can delete this warning once\nyou add code to this MHL case"
            # "Workers Public API Request Case"
            n96 = Variant To Data(error in=w208, type=T22 {"String"=""} ("Data"), Variant=w205) -> (data=w204:T22, error out=w207:errorcluster)
            n97 = Unbundle By Name(w204) -> ()  [unwired: 1 out]
            n98 = Merge Errors(w207) -> (w203:errorcluster)
          }
          frame "Get Initialize Data" {
            # "Workers Public API Request Case"
            n99 = Variant To Data(error in=w215, type=T23 {"Дата"="", "Время"="", "Месторождение"="", "Пласт"="", "Скважина"=""} ("Data"), Variant=w212) -> (data=w211:T23, error out=w214:errorcluster)
            n100 = Unbundle By Name(w211) -> ()  [unwired: 5 out]
            n101 = Merge Errors(w214) -> (w210:errorcluster)
          }
          frame "Write CMD" {
            # "Workers Public API Request Case"
            n102 = Variant To Data(error in=w232, type=T24 {"CMD"={"Rotate_CMD"=0, "Termex_CMD"=0, "Mix_CMD"=0, "Rotate_SP_Angle_Init"=0, "Rotate_SP_Angle_End"=0, "Rotate_SP_Timeout"=0, "Rotate_SP_Speed"=0, "T_SP"=0.0, "KP"=0.0, "TN"=0.0, "Mix_SP"=0}} ("Data"), Variant=w230) -> (data=w229:T24, error out=w227:errorcluster)
            n103 = Unbundle By Name(w225) -> ("Modbus PLC"=w224:refnum<class "Modbus PLC.lvclass">, "Heater"=w221:cluster{"P":dbl, "I":dbl})
            n104 = Unbundle By Name(w229) -> ("CMD"=w220:T3)
            n105 = Unbundle By Name(w221) -> ("P"=w219:dbl, "I"=w218:dbl)
            n106 = Bundle By Name(cluster=w220, "KP"=w219, "TN"=w218) -> (w217:T3)
            n107 = call-dynamic "rqp_Write.vi"("Caller in"=w225, "error in"=w227, "Data in"=w217, "Base Hardware in"=w224) -> ("error out"=w226:errorcluster, "dup Base Hardware out"=w222:refnum<class "Modbus PLC.lvclass">)  [unwired: 6 in]
            n108 = Bundle By Name(cluster=w225, "Modbus PLC"=w222) -> (w223:refnum<class "gui.lvclass">)
            n109 = Merge Errors(w226) -> (w228:errorcluster)
          }
          frame "------------- RESPONSE CASES --------------" {
            # "Start of Workers Response Cases"
          }
          frame "Get Settings" {
            # "This case receives a Response message from a subWorker"
            n110 = call "rspvtd_Get Settings.vi"("error in"=w266, "Data in"=w267) -> ("error out"=w257:errorcluster, "Data out"=w248:T29)  [unwired: 8 in]
            n111 = Unbundle(w248) -> ("Settings"=w263:T30)
            n112 = Unbundle By Name(w248) -> ("Settings.PLC1"=w254:cluster{"port":u16, "address":string})
            n113 = Unbundle By Name(w263) -> ("PLC2.address"=w260:string, "PLC2.port"=w259:u16)
            n114 = control-ref of="Насос"() -> (w249:refnum<vi>)
            n115 = control-ref of="Насос 2"() -> (w250:refnum<vi>)
            n116 = control-ref of="Насосная система"() -> (w251:refnum<vi>)
            n117 = control-ref of="Параметры"() -> (w252:refnum<vi>)
            n118 = Bundle By Name(cluster=w265, "Settings"=w263) -> (w256:refnum<class "gui.lvclass">)
            n119 = Unbundle By Name(w254) -> ("address"=w253:string)
            n120 = Bundle("address"=w260, "port"=w259) -> (w258:cluster{"address":string, "port":u16})  [unwired: 1 in]
            n121 = Bundle By Name(cluster=T25 {"Pump"=refnum, "Params"=refnum, "Pump2"=refnum, "Pump System"=refnum, "IP Adress"=""} ("Data in"), "Pump"=w249, "Pump2"=w250, "Pump System"=w251, "Params"=w252, "IP Adress"=w253) -> (w240:T25)
            n122 = Unbundle By Name(w256) -> ("Modbus PLC"=w239:refnum<class "Modbus PLC.lvclass">, "Pumps Worker"=w255:refnum<class "Pumps Worker.lvclass">)
            n123 = call "rqp_Stop Session.vi"("Caller in"=w256, "error in"=w257, "Pumps Worker in"=w255) -> ("error out"=w246:errorcluster, "dup Pumps Worker out"=w242:refnum<class "Pumps Worker.lvclass">, "dup Caller out"=w243:refnum<class "gui.lvclass">)  [unwired: 6 in]
            n124 = call "rqp_Get Settings.vi"("Caller in"=w243, "error in"=w246, "Data in"=w240, "Pumps Worker in"=w242) -> ("error out"=w247:errorcluster, "dup Pumps Worker out"=w241:refnum<class "Pumps Worker.lvclass">, "dup Caller out"=w238:refnum<class "gui.lvclass">)  [unwired: 5 in]
            n125 = call "rqp_Start Session.vi"("error in"=w247, "Pumps Worker in"=w241) -> ("error out"=w235:errorcluster, "dup Pumps Worker out"=w245:refnum<class "Pumps Worker.lvclass">)  [unwired: 7 in, 1 out]
            n126 = call-dynamic "rqp_Close.vi"("Caller in"=w238, "error in"=w235, "Base Hardware in"=w239) -> ("error out"=w236:errorcluster, "dup Base Hardware out"=w237:refnum<class "Modbus PLC.lvclass">)  [unwired: 7 in]
            n127 = call-dynamic "rqp_Init.vi"("Caller in"=w238, "error in"=w236, "Data in"=w258, "Base Hardware in"=w237) -> ("error out"=w264:errorcluster, "dup Base Hardware out"=w262:refnum<class "Modbus PLC.lvclass">)  [unwired: 6 in]
            n128 = Merge Errors(w264) -> (w268:errorcluster)
            n129 = Bundle By Name(cluster=w238, "Modbus PLC"=w262, "Pumps Worker"=w245) -> (w261:refnum<class "gui.lvclass">)
          }
          frame "Update Data" {
            # "This case receives a Response message from a subWorker"
            n130 = local read "Насосная система"() -> (w269:T2)
            n131 = Unbundle By Name(w269) -> ()  [unwired: 3 out]
            n132 = Merge Errors(w272) -> (w270:errorcluster)
          }
          frame "New Pumps Data" {
            # "This case receives a Response message from a subWorker"
            n133 = call "rspvtd_New Pumps Data.vi"("error in"=w279, "Data in"=w280) -> ("error out"=w278:errorcluster, "Data out"=w277:T31)  [unwired: 8 in]
            n134 = Unbundle By Name(w277) -> ("Насос"=w276:T7, "Насос 2"=w275:T6, "Насосная система"=w274:T2)
            n135 = local write "Насос"(w276) -> ()
            n136 = local write "Насос 2"(w275) -> ()
            n137 = local write "Насосная система"(w274) -> ()
            n138 = Merge Errors(w278) -> (w273:errorcluster)
          }
          frame "Starting Settings" {
            # "This case receives a Response message from a subWorker"
            n139 = call "rspvtd_Starting Settings.vi"("error in"=w309, "Data in"=w308) -> ("error out"=w306:errorcluster, "Data out"=w307:T32)  [unwired: 8 in]
            n140 = Unbundle(w307) -> ("Settings"=w303:T30)
            n141 = Unbundle By Name(w305) -> ("Pumps Worker"=w292:refnum<class "Pumps Worker.lvclass">, "Modbus PLC"=w289:refnum<class "Modbus PLC.lvclass">)
            n142 = Unbundle By Name(w303) -> ("PLC1"=w301:cluster{"port":u16, "address":string}, "PLC2"=w286:cluster{"port":u16, "address":string})
            n143 = control-ref of="Насос"() -> (w296:refnum<vi>)
            n144 = control-ref of="Насос 2"() -> (w297:refnum<vi>)
            n145 = control-ref of="Насосная система"() -> (w298:refnum<vi>)
            n146 = control-ref of="Параметры"() -> (w299:refnum<vi>)
            n147 = Unbundle By Name(w301) -> ("address"=w300:string)
            n148 = Bundle By Name(cluster=T25 {"Pump"=refnum, "Params"=refnum, "Pump2"=refnum, "Pump System"=refnum, "IP Adress"=""} ("Data in"), "Pump"=w296, "Pump2"=w297, "Pump System"=w298, "Params"=w299, "IP Adress"=w300) -> (w295:T25)
            n149 = call "rqp_Get Settings.vi"("Caller in"=w305, "error in"=w306, "Data in"=w295, "Pumps Worker in"=w292) -> ("error out"=w293:errorcluster, "dup Pumps Worker out"=w285:refnum<class "Pumps Worker.lvclass">, "dup Caller out"=w294:refnum<class "gui.lvclass">)  [unwired: 5 in]
            n150 = call "rqp_Start Session.vi"("Caller in"=w294, "error in"=w293, "Pumps Worker in"=w285) -> ("error out"=w291:errorcluster, "dup Pumps Worker out"=w284:refnum<class "Pumps Worker.lvclass">, "dup Caller out"=w288:refnum<class "gui.lvclass">)  [unwired: 6 in]
            n151 = call-dynamic "rqp_Init.vi"("Message Priority"=Priority."High", "Caller in"=w288, "error in"=w291, "Data in"=w286, "Base Hardware in"=w289) -> ("error out"=w290:errorcluster, "dup Base Hardware out"=w287:refnum<class "Modbus PLC.lvclass">)  [unwired: 5 in]
            n152 = Bundle By Name(cluster=w288, "Pumps Worker"=w284, "Modbus PLC"=w287) -> (w304:refnum<class "gui.lvclass">)
            n153 = Merge Errors(w290) -> (w282:errorcluster)
          }
          frame "Data From PLC" {
            # "This case receives a Response message from a subWorker"
            n154 = Variant To Data(error in=w334, type=T4 {"Rotate_IND"=0, "Termex_IND"=0, "Mix_IND"=0, "Rotate_PV_Angle_Init"=0, "Rotate_PV_Angle_End"=0, "Rotate_PV_Timeout"=0, "Rotate_PV_Speed"=0, "Rotate_PV_Time"=0, "Rotate_PV_Angle"=0, "Termex_SP"=0.0, "MIX_PV"=0, "Termex_PV_In"=0.0, "Termex_KP"=0.0, "P_PV"=0.0, "Termex_PV_Out"=0.0, "Termex_TN"=0.0, "MM_PV"=0.0} ("IND"), Variant=w331) -> (data=w317:T4, error out=w333:errorcluster)
            "data" <- w317
            n155 = Unbundle By Name(w330) -> ("Calcs"=w324:T33)
            n156 = Unbundle By Name(w317) -> ("MM_PV"=w327:sgl)
            n157 = local read "Current Temperature"() -> (w328:dbl)
            n158 = property on="Давление в системе" class="DigNum (strict)"() -> ("Value"=w329:dbl)  [unwired: 2 in, 2 out]
            n159 = call "Calcs.vi"("h"=w327, "T"=w328, "P"=w329, "Calcs"=w324) -> ("Vcorr"=→"V ind":dbl)  [unwired: 5 in, 2 out]
            n160 = Unbundle By Name(w317) -> ("Termex_PV_In"=w316:sgl, "Termex_PV_Out"=w314:sgl, "P_PV"=→"P ind":sgl)
            "T ind" <- w314
            n161 = control-ref of="Rotate"() -> (w325:refnum<vi>)
            n162 = control-ref of="Скорость, об/мин"() -> (w323:refnum<vi>)
            n163 = control-ref of="Mixer Start"() -> (w322:refnum<vi>)
            n164 = control-ref of="Уставка, °С"() -> (w320:refnum<vi>)
            n165 = control-ref of="Heater Start Btn"() -> (w319:refnum<vi>)
            n166 = local write "Termostat"(w316) -> ()
            n167 = local write "Current Temperature"(w314) -> ()
            n168 = call "Get Rotate Data.vi"("IND"=w317, "Rotate Ref"=w325) -> ("error out"=w321:errorcluster)  [unwired: 9 in]
            n169 = call "Get Mixer.vi"("error in (no error)"=w321, "Mix Btn Ref"=w322, "Speed Ref"=w323, "data"=w317) -> ("error out"=w318:errorcluster)  [unwired: 7 in]
            n170 = call "Get Heater.vi"("error in (no error)"=w318, "Heater Start Btn"=w319, "Digital in"=w320, "data"=w317) -> ("error out"=w312:errorcluster)  [unwired: 7 in]
            n171 = Generate User Event(user event=w313, event data cluster=variant ("event data"), error in=w312) -> (error out=w311:errorcluster)  [unwired: 1 in, 1 out]
            n172 = Merge Errors(w311, w333) -> (w335:errorcluster)
          }
          frame "Update Reg Status" {
            # "This case receives a Response message from a subWorker"
            n173 = call "rspvtd_Record Status to Caller.vi"("error in"=w339, "Data in"=w337) -> ("error out"=w338:errorcluster, "Data out"=w336:T34)  [unwired: 8 in]
            n174 = property on="Registration Btn" class="Bool"("Value"=w336) -> ()  [unwired: 2 in, 2 out]
            n175 = Merge Errors(w338) -> (w340:errorcluster)
          }
        }
        n176 = call-dynamic "Error Handler.vi"("Worker"=w68, "error_in"=w70) -> ("error out"=w73:errorcluster, "Stop Loop"=w66:bool, "Worker out"=w72:refnum<class "gui.lvclass">)  [unwired: 7 in]
      }
      n177 = call-dynamic "Setup EHL.vi"("Worker"=w57) -> ("Worker out"=w58:refnum<class "gui.lvclass">)  [unwired: 14 in]
      n178 = while "Event Handling Loop" {
        shift-right: [w354] -> w61
        shift-left: w62 -> [w353]
        tunnel: [w349] -> w59
        tunnel: errorcluster {"status"=FALSE, "code"=0, "source"=""} ("error constant") -> [w351]
        shift-right: [w347] -> _
        shift-left: w58 -> [w352]
        tunnel: w54 -> [w345]
        shift-right: [w343] -> _
        shift-left: "CMD" -> [w344]
        tunnel: w51 -> [w342]
        stop <- w346 stop-if-true
        # "Event Handling Loop"
        n179 = event shown="[1] \"Registration Btn\": Value Change" {
          selector: w353 -> [_ _ _ _ _ _ _ _ _ _ _ _ _ _ _ _ _]
          dyn-events: [_ _ _ _ _ _ _ _ _ _ _ _ _ _ _ _ _] -> w354
          timeout: _ -> [_ _ _ _ _ _ _ _ _ _ _ _ _ _ _ _ _]
          tunnel: [w359 w364 w371 w375 w382 w385 w388 w391 w396 w399 w406 w412 w426 w439 w445 w456 w481] -> w350
          tunnel: w351 -> [w360 w364 w370 w375 w382 w385 w388 w391 w396 w400 w407 w413 w427 w440 w446 w457 w481]
          tunnel: w352 -> [w358 w361 w369 w374 w381 w384 w387 w390 w395 w402 w408 w417 w429 w442 w447 w461 w497]
          tunnel: [w357 w361 w368 w374 w381 w384 w387 w390 w395 w401 w408 w416 w428 w441 w443 w460 w497] -> w348
          tunnel: w345 -> [_ _ _ _ _ _ _ _ _ _ w405 _ _ _ _ _ _]
          tunnel: w344 -> [w355 w363 w365 w373 w376 w383 w386 w389 w392 w397 w403 w425 w437 w438 w444 w479 w517]
          tunnel: [w355 w363 w365 w373 w376 w383 w386 w389 w392 w397 w403 w415 w430 w438 w444 w459 w499] -> w343
          tunnel: w342 -> [_ w362 _ _ _ _ _ _ _ _ _ _ _ _ _ _ _]
          event User Event {
            # "This case and its contents must always be included in every EHL that you use, so that the framework can automatically stop the EHL."
            # "EHL Stop Event. This EHL exits from this case."
            n180 = event-data() -> ("Stop Event Data"=w356:variant)  [unwired: 1 in]
            n181 = call-dynamic "EHL Stop - EHL Case.vi"("error in"=w360, "Stop Event Data"=w356, "Worker"=w358) -> ("error out"=w359:errorcluster, "Worker out"=w357:refnum<class "gui.lvclass">)  [unwired: 7 in]
          }
          event "Registration Btn": Value Change {
            n182 = event-data() -> ()  [unwired: 1 in, 4 out]
            n183 = call "rqp_Show UI.vi"("Caller in"=w361, "Registration in"=w362) -> ()  [unwired: 7 in, 3 out]
          }
          event Panel Close? {
            # "Use this VI when you want to exit this Worker. This VI will call the Start Exiting case of this Worker. This is the correct way to exit your Worker."
            # "Calls the Start Exiting case of this Worker. This will start the exiting sequence of this Worker."
            n184 = event-data() -> ()  [unwired: 1 in, 1 out]
            n185 = property class="gui"(reference=w369) -> (reference out=w367:refnum<class "gui.lvclass">, "Accessors:Read:Public API:Queue"=w366:refnum<class "Message Queue.lvclass">)  [unwired: 1 in, 1 out]
            n186 = call-dynamic "Worker Start Exiting.vi"("error_in"=w370, "Message Queue"=w366, "Worker"=w367) -> ("error out"=w371:errorcluster, "dup Worker out"=w368:refnum<class "gui.lvclass">)  [unwired: 7 in]
            n187 = event-data ("Event Filter Node")("Discard?"=TRUE) -> ()  [unwired: 1 in, 1 out]
          }
          event "CurvePV Btn": Value Change {
            n188 = event-data() -> ()  [unwired: 1 in, 1 out]
            n189 = call "Show Panel.vi"() -> ()  [unwired: 11 in, 1 out]
          }
          event User Event {
            n190 = event-data() -> ("Temp Variation By Speed"=w378:bool)  [unwired: 1 in]
            n191 = Select(t=T27."Enabled" ("Disabled"), s=w378, f=T27."Disabled and Grayed Out" ("Disabled")) -> (s? t:f=w377:T27)
            n192 = property on="End by temperature" class="DigNum (strict)"("DisabledEnum"=w377) -> ()  [unwired: 2 in, 2 out]
            n193 = property on="Temp speed" class="DigNum (strict)"("DisabledEnum"=w377) -> ()  [unwired: 2 in, 2 out]
          }
          event "Camera Btn": Value Change {
            n194 = event-data() -> ()  [unwired: 1 in, 6 out]
          }
          event "Control Button": Value Change {
            n195 = event-data() -> ()  [unwired: 1 in, 6 out]
          }
          event "Graph Btn": Value Change {
            n196 = event-data() -> ()  [unwired: 1 in, 1 out]
            n197 = call "Show Panel.vi"() -> ()  [unwired: 11 in, 1 out]
          }
          event User Event {
            n198 = event-data() -> ("VI Refnum"=w394:refnum<vi>)  [unwired: 1 in]
            n199 = control-ref of="Sub Panel"() -> (w393:refnum<vi>)
            n200 = call "Insert SubPanel.vi"("VI Ref"=w394, "Subpanel Ref"=w393) -> ()  [unwired: 9 in, 1 out]
          }
          event User Event {
            n201 = event-data() -> ("Исходные данные"=w398:T35)  [unwired: 1 in]
            n202 = call "rqp_Get Initialize Data.vi"("error in"=w400, "Data in"=w398, "gui in"=w402) -> ("error out"=w399:errorcluster, "dup gui out"=w401:refnum<class "gui.lvclass">)  [unwired: 6 in, 1 out]
          }
          event "Temp Speed Mode": Value Change {
            n203 = event-data() -> ("NewVal"=w404:bool)  [unwired: 1 in]
            n204 = Generate User Event(user event=w405, event data cluster=w404, error in=w407) -> (error out=w406:errorcluster)  [unwired: 1 in, 1 out]
          }
          event "Mixer Start", "Скорость, об/мин": Value Change {
            w419 = u16 9 items=["Мешалка движение вперёд"=1, "Мешалка движение назад"=2, "Мешалка стоп"=9] ("Mix_CMD")
            w422 = u16 2 items=["Мешалка движение вперёд"=1, "Мешалка движение назад"=2, "Мешалка стоп"=9] ("Mix_CMD")
            w423 = u16 1 items=["Мешалка движение вперёд"=1, "Мешалка движение назад"=2, "Мешалка стоп"=9] ("Mix_CMD")
            n205 = event-data() -> ()  [unwired: 1 in, 1 out]
            n206 = Less Than 0?(x="Скорость, об/мин") -> (x < 0?=w424:bool)
            n207 = Absolute Value(x="Скорость, об/мин") -> (abs(x)=w410:dbl)
            n208 = Select(t=w422, s=w424, f=w423) -> (s? t:f=w420:u16)
            n209 = To Unsigned Word Integer(number=w410) -> (unsigned 16bit integer=w409:u16)
            n210 = Select(t=w420, s="Mixer Start", f=w419) -> (s? t:f=w418:u16)
            n211 = Bundle By Name(cluster=w425, "Mix_CMD"=w418, "Mix_SP"=w409) -> (w415:T3)
            n212 = Bundle("CMD"=w415) -> (w414:cluster{"CMD":T3})  [unwired: 1 in]
            n213 = call "rqp_Write CMD.vi"("error in"=w413, "Data in"=w414, "gui in"=w417) -> ("error out"=w412:errorcluster, "dup gui out"=w416:refnum<class "gui.lvclass">)  [unwired: 6 in, 1 out]
          }
          event "Heater Start Btn", "Уставка, °С": Value Change {
            w435 = u16 9 items=["Термостат старт"=1, "Термостат стоп"=9] ("Termex_CMD")
            w436 = u16 1 items=["Термостат старт"=1, "Термостат стоп"=9] ("Termex_CMD")
            n214 = event-data() -> ()  [unwired: 1 in, 1 out]
            n215 = Select(t=w436, s="Heater Start Btn", f=w435) -> (s? t:f=w433:u16)
            n216 = Bundle By Name(cluster=w437, "Termex_CMD"=w433, "T_SP"="Уставка, °С") -> (w430:T3)
            n217 = Bundle("CMD"=w430) -> (w431:cluster{"CMD":T3})  [unwired: 1 in]
            n218 = call "rqp_Write CMD.vi"("error in"=w427, "Data in"=w431, "gui in"=w429) -> ("error out"=w426:errorcluster, "dup gui out"=w428:refnum<class "gui.lvclass">)  [unwired: 6 in, 1 out]
          }
          event "Settings Btn": Value Change {
            n219 = event-data() -> ()  [unwired: 1 in, 1 out]
            n220 = call "rqp_Open Settings.vi"("error in"=w440, "gui in"=w442) -> ("error out"=w439:errorcluster, "dup gui out"=w441:refnum<class "gui.lvclass">)  [unwired: 7 in, 1 out]
          }
          event Value Change {
            n221 = event-data() -> ()  [unwired: 1 in, 1 out]
            n222 = disable-structure shown="Enabled" {
              disable-tunnel: w447 -> [w451 w455]
              disable-tunnel: w446 -> [w450 w453]
              disable-tunnel: [w449 w452] -> w445
              disable-tunnel: [w448 w454] -> w443
              frame Disabled {
                n223 = call "rql_Push Pumps.vi"("error in"=w450, "gui in"=w451) -> ("error out"=w449:errorcluster, "dup gui out"=w448:refnum<class "gui.lvclass">)  [unwired: 8 in]
              }
              frame Enabled {
                n224 = call "rqp_Pumps Change.vi"("error in"=w453, "gui in"=w455) -> ("error out"=w452:errorcluster, "dup gui out"=w454:refnum<class "gui.lvclass">)  [unwired: 7 in, 1 out]
              }
            }
          }
          event Value Change {
            w469 = u16 1 items=["Качалка Дом"=1, "Качалка Режим Авто - Старт"=2, "Качалка Режим Ручной - Старт"=3, "Качалка Стоп"=9] ("Rotate_CMD")
            w472 = u16 9 items=["Качалка Дом"=1, "Качалка Режим Авто - Старт"=2, "Качалка Режим Ручной - Старт"=3, "Качалка Стоп"=9] ("Rotate_CMD")
            w473 = u16 2 items=["Качалка Дом"=1, "Качалка Режим Авто - Старт"=2, "Качалка Режим Ручной - Старт"=3, "Качалка Стоп"=9] ("Rotate_CMD")
            w476 = u16 3 items=["Качалка Дом"=1, "Качалка Режим Авто - Старт"=2, "Качалка Режим Ручной - Старт"=3, "Качалка Стоп"=9] ("Rotate_CMD")
            n225 = event-data() -> ("NewVal"=w480:T1)  [unwired: 1 in]
            n226 = Unbundle By Name(w480) -> ("Mode"=w464:u16, "SP_Angle"=w467:dbl, "Rotate Angle"=w468:dbl, "Timeout"=w475:dbl, "Start"=w474:bool, "Home"=w471:bool)  [unwired: 1 out]
            n227 = Equal?(x=u16 1 ("y"), y=w464) -> (x = y?=w477:bool)
            n228 = To Unsigned Word Integer(number=w468) -> (unsigned 16bit integer=w466:u16)
            n229 = Select(t=w476, s=w477, f=w473) -> (s? t:f=w463:u16)
            n230 = Select(t=w463, s=w474, f=w472) -> (s? t:f=w470:u16)
            n231 = Select(t=w469, s=w471, f=w470) -> (s? t:f=w462:u16)
            n232 = Bundle By Name(cluster=w479, "Rotate_CMD"=w462, "Rotate_SP_Timeout"=w475, "Rotate_SP_Angle_Init"=w467, "Rotate_SP_Angle_End"=w466, "Rotate_SP_Speed"=u16 50) -> (w459:T3)
            n233 = Bundle("CMD"=w459) -> (w458:cluster{"CMD":T3})  [unwired: 1 in]
            n234 = call "rqp_Write CMD.vi"("error in"=w457, "Data in"=w458, "gui in"=w461) -> ("error out"=w456:errorcluster, "dup gui out"=w460:refnum<class "gui.lvclass">)  [unwired: 6 in, 1 out]
          }
          event User Event {
            w488 = u16 9 items=["Мешалка движение вперёд"=1, "Мешалка движение назад"=2, "Мешалка стоп"=9] ("Mix_CMD")
            w486 = u16 2 items=["Мешалка движение вперёд"=1, "Мешалка движение назад"=2, "Мешалка стоп"=9] ("Mix_CMD")
            w487 = u16 1 items=["Мешалка движение вперёд"=1, "Мешалка движение назад"=2, "Мешалка стоп"=9] ("Mix_CMD")
            w495 = u16 9 items=["Термостат старт"=1, "Термостат стоп"=9] ("Termex_CMD")
            w496 = u16 1 items=["Термостат старт"=1, "Термостат стоп"=9] ("Termex_CMD")
            w507 = u16 1 items=["Качалка Дом"=1, "Качалка Режим Авто - Старт"=2, "Качалка Режим Ручной - Старт"=3, "Качалка Стоп"=9] ("Rotate_CMD")
            w510 = u16 9 items=["Качалка Дом"=1, "Качалка Режим Авто - Старт"=2, "Качалка Режим Ручной - Старт"=3, "Качалка Стоп"=9] ("Rotate_CMD")
            w511 = u16 2 items=["Качалка Дом"=1, "Качалка Режим Авто - Старт"=2, "Качалка Режим Ручной - Старт"=3, "Качалка Стоп"=9] ("Rotate_CMD")
            w514 = u16 3 items=["Качалка Дом"=1, "Качалка Режим Авто - Старт"=2, "Качалка Режим Ручной - Старт"=3, "Качалка Стоп"=9] ("Rotate_CMD")
            n235 = event-data() -> ()  [unwired: 1 in, 1 out]
            n236 = Unbundle By Name("Rotate") -> ("Mode"=w502:u16, "SP_Angle"=w505:dbl, "Rotate Angle"=w506:dbl, "Timeout"=w513:dbl, "Start"=w512:bool, "Home"=w509:bool)  [unwired: 1 out]
            n237 = local read "Heater Start Btn"() -> (w494:bool)
            n238 = Equal?(x=u16 1 ("y"), y=w502) -> (x = y?=w515:bool)
            n239 = To Unsigned Word Integer(number=w506) -> (unsigned 16bit integer=w504:u16)
            n240 = Select(t=w496, s=w494, f=w495) -> (s? t:f=w492:u16)
            n241 = local read "Скорость, об/мин"() -> (w484:dbl)
            n242 = local read "Уставка, °С"() -> (w493:sgl)
            n243 = local read "Mixer Start"() -> (w485:bool)
            n244 = Absolute Value(x=w484) -> (abs(x)=w489:dbl)
            n245 = Less Than 0?(x=w484) -> (x < 0?=w491:bool)
            n246 = Select(t=w486, s=w491, f=w487) -> (s? t:f=w490:u16)
            n247 = To Unsigned Word Integer(number=w489) -> (unsigned 16bit integer=w482:u16)
            n248 = Select(t=w514, s=w515, f=w511) -> (s? t:f=w501:u16)
            n249 = Select(t=w501, s=w512, f=w510) -> (s? t:f=w508:u16)
            n250 = Select(t=w507, s=w509, f=w508) -> (s? t:f=w500:u16)
            n251 = Select(t=w490, s=w485, f=w488) -> (s? t:f=w483:u16)
            n252 = Bundle By Name(cluster=w517, "Rotate_CMD"=w500, "Rotate_SP_Timeout"=w513, "Rotate_SP_Angle_Init"=w505, "Rotate_SP_Angle_End"=w504, "Rotate_SP_Speed"=u16 50, "T_SP"=w493, "Termex_CMD"=w492, "Mix_CMD"=w483, "Mix_SP"=w482) -> (w499:T3)
          }
        }
        n253 = call-dynamic "Error Handler.vi"("Worker"=w348, "error_in"=w350) -> ("error out"=w349:errorcluster, "Stop Loop"=w346:bool, "Worker out"=w347:refnum<class "gui.lvclass">)  [unwired: 7 in]
      }
    }
    frame Error {
      n254 = call-dynamic "Error Handler.vi"("Worker"=w519, "error_in"=w522) -> ("error out"=w520:errorcluster, "Worker out"=w518:refnum<class "gui.lvclass">)  [unwired: 7 in, 1 out]
    }
  }
  n255 = call-dynamic "Main.vi"("error in"=w17, "Pumps Worker in"=w8) -> ("error out"=w10:errorcluster)  [unwired: 8 in, 1 out]
  n256 = call-dynamic "Main.vi"("error in"=w17, "Modbus PLC in"=w6) -> ("error out"=w7:errorcluster)  [unwired: 8 in, 1 out]
  n257 = call-dynamic "Main.vi"("error in"=w17, "Registration in"=w1) -> ("error out"=w2:errorcluster)  [unwired: 8 in, 1 out]
  n258 = Merge Errors(w10, w7, w2) -> (w9:errorcluster)
  n259 = Unregister For Events(event registration refnum=w48, error in=w49) -> (error out=w50:errorcluster)
  n260 = Merge Errors(w50, w45, w9) -> (w47:errorcluster)
  n261 = call-dynamic "Exited Notify and Cleanup.vi"("error_in"=w47, "Worker"=w46) -> ("error out"=→"error out":errorcluster, "dup Worker out"=→"gui out":refnum<class "gui.lvclass">)  [unwired: 8 in]
